vi "Generate Text Report.vi"(8 "error in (no error)":errorcluster, 11 "XML Report In":refnum<class "XML Report.lvclass">) -> (0 "error out":errorcluster, 2 "XML":string, 3 "XML Report Out":refnum<class "XML Report.lvclass">)   [LabVIEW 2020, in "XML Report.lvclass"]
uses:
  XML Report.lvclass
  Test Report/Test Report.lvclass
  <vilib>/xml/NI_XML.lvlib
  <resource>/objmgr/DOMUserDefRef.rc
  <vilib>/xml/Close Reference(Node).vi
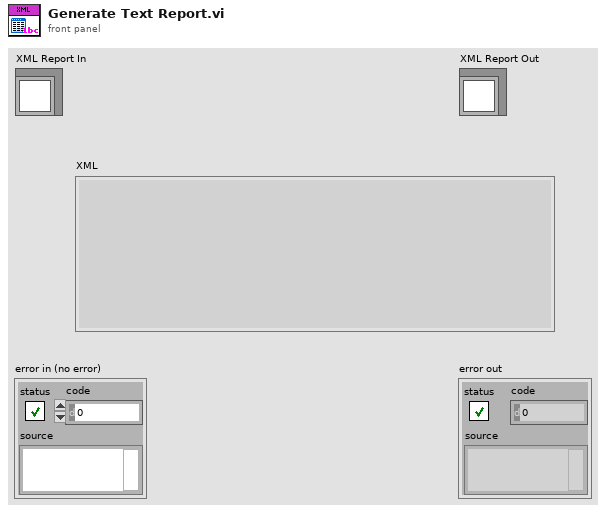
[diagram p1: front panel]
types:
  T1 = typedef "Test Suite Result.lvlib/Test Suite Result.ctl" = cluster{"Test Suite ID":string, "Name":string, "Hostname":string, "Status":T2, "Execution time":dbl, "Start Time":timestamp, "Case Results":T3[]}
  T2 = typedef "Assertion Result.lvlib/Status.ctl" = enum16{"Pass", "Fail", "Error", "Skipped", "Setup Error", "Broken", "Teardown Error"}
  T3 = typedef "Test Case Result.lvlib/Test Case Result.ctl" = map{string, T4}
  T4 = typedef "Method Result.lvlib/Method Result.ctl" = cluster{"Test Case":string, "Test Method Name":string, "Status":T2, "Assertion Results":T5[], "Execution time":dbl, "Result String":string}
  T5 = typedef "Assertion Result.lvlib/Assertion Result.ctl" = cluster{"Status":T2, "Message":string, "Description":string, "Assertion Type":T6}
  T6 = typedef "Assertion Result.lvlib/Assertion Type.ctl" = enum16{"None", "Pass", "Fail", "Skip", "Pass if Equal", "Fail if Equal", "Pass if Error", "Fail if Error", "Pass if", "Fail if"}
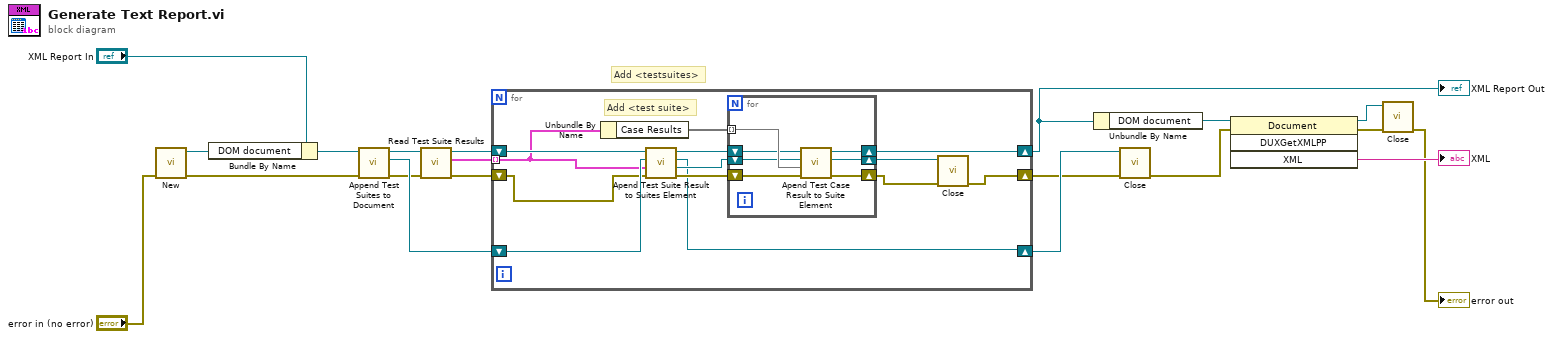
[diagram p0: block diagram]
diagram:
  # "Add <testsuites>"
  n1 = call <vilib>:"New.vi"("error in (no error)"="error in (no error)") -> ("error out"=w20:errorcluster, "DOM document out"=w17:refnum<k20>)  [unwired: 7 in]
  n2 = Bundle By Name(cluster="XML Report In", "DOM document"=w17) -> (w15:refnum<class "XML Report.lvclass">)
  n3 = call "Append Test Suites to Document.vi"("error in (no error)"=w20, "XML Report In"=w15) -> ("error out"=w2:errorcluster, "Test Suites Element"=w19:refnum<k20>, "XML Report Out"=w4:refnum<class "XML Report.lvclass">)  [unwired: 7 in]
  n4 = call "Read Test Suite Results.vi"("error in (no error)"=w2, "Report In"=w4) -> ("error out"=w1:errorcluster, "Test Suite Results"=w5:T1[], "Report Out"=w3:refnum<class "XML Report.lvclass">)  [unwired: 7 in]
  n5 = for {
    tunnel: w5 -> [w21] mode=indexing
    shift-right: [w27] -> w7
    shift-left: w1 -> [w23]
    shift-right: [w26] -> w13
    shift-left: w3 -> [w33]
    shift-right: [w24] -> w8
    shift-left: w19 -> [w31]
    # "Add <test suite>"
    n6 = Unbundle By Name(w21) -> ("Case Results"=w22:T3[])
    n7 = call "Apend Test Suite Result to Suites Element.vi"("error in (no error)"=w23, "Test Suite Result"=w21, "Test Suites Element in"=w31, "XML Report In"=w33) -> ("error out"=w25:errorcluster, "Test Suite Element"=w30:refnum<k20>, "Test Suites Element out"=w24:refnum<k20>, "XML Report Out"=w32:refnum<class "XML Report.lvclass">)  [unwired: 4 in]
    n8 = for {
      tunnel: w22 -> [w39] mode=indexing
      shift-right: [w37] -> w28
      shift-left: w30 -> [w38]
      shift-right: [w35] -> w29
      shift-left: w25 -> [w40]
      shift-right: [w34] -> w26
      shift-left: w32 -> [w36]
      n9 = call "Apend Test Case Result to Suite Element.vi"("error in (no error)"=w40, "Test Case Result"=w39, "Test Suite Element in"=w38, "XML Report In"=w36) -> ("error out"=w35:errorcluster, "Test Suite Element out"=w37:refnum<k20>, "XML Report Out"=w34:refnum<class "XML Report.lvclass">)  [unwired: 5 in]
    }
    n10 = call-poly <vilib>:"Close.vi"("error in (no error)"=w29, "node"=w28) -> ("error out"=w27:errorcluster)  [unwired: 7 in]
  }
  "XML Report Out" <- w13
  n11 = Unbundle By Name(w13) -> ("DOM document"=w12:refnum<k20>)
  n12 = call-poly <vilib>:"Close.vi"("error in (no error)"=w7, "node"=w8) -> ("error out"=w6:errorcluster)  [unwired: 7 in]
  n13 = invoke class="Document" method="DUXGetXMLPP"(reference=w12, error in=w6) -> (reference out=w10:refnum<k20>, error out=w11:errorcluster, "XML"=→"XML":string)  [unwired: 2 in, 1 out]
  n14 = call-poly <vilib>:"Close.vi"("error in (no error)"=w11, "node"=w10) -> ("error out"=→"error out":errorcluster)  [unwired: 7 in]
